vi "比较-日期时间组合数组.vi"(8 "比较模式":enum16{"A>B?", "A<B?", "A>=B?", "A<=B?", "A=B?"}(ring), 10 "日期时间B":i32[](array[numeric]), 11 "日期时间A":i32[](array[numeric])) -> (3 "结果":bool)   [LabVIEW 2013]
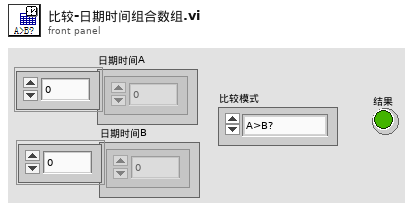
[diagram p1: front panel]
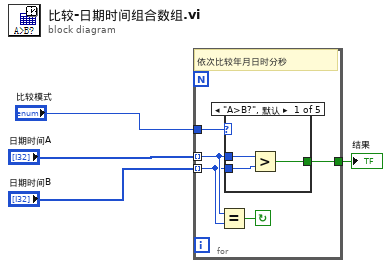
[diagram p0: block diagram]
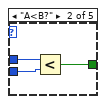
[diagram p2: hidden frame]
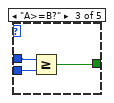
[diagram p3: hidden frame]
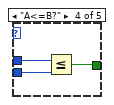
[diagram p4: hidden frame]
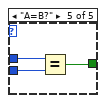
[diagram p5: hidden frame]
diagram:
  n1 = for {
    tunnel: "日期时间A" -> [w8] mode=indexing
    tunnel: "日期时间B" -> [w7] mode=indexing
    tunnel: "比较模式" -> [w6]
    tunnel: [w5] -> w1
    stop <- w9 continue-if-true
    # "依次比较年月日时分秒"
    n2 = Equal?(x=w8, y=w7) -> (x = y?=w9:bool)
    n3 = case shown="\"A>B?\", 默认" w6 {
      tunnel: w8 -> [w12 w15 w17 w20 w23]
      tunnel: w7 -> [w11 w14 w18 w19 w22]
      tunnel: [w10 w13 w16 w21 w24] -> w5
      frame "A>B?", Default {
        n4 = Greater?(x=w12, y=w11) -> (0:w10:bool)
      }
      frame "A<B?" {
        n5 = Less?(x=w15, y=w14) -> (x < y?=w13:bool)
      }
      frame "A>=B?" {
        n6 = Greater Or Equal?(x=w17, y=w18) -> (x >= y?=w16:bool)
      }
      frame "A<=B?" {
        n7 = Less Or Equal?(x=w20, y=w19) -> (x <= y?=w21:bool)
      }
      frame "A=B?" {
        n8 = Equal?(x=w23, y=w22) -> (x = y?=w24:bool)
      }
    }
  }
  "结果" <- w1
